vi "Get Fault States.vi"(8 "error in (no error)":errorcluster, 11 "FIU Board Ref in":T1 format="%.0x") -> (0 "error out":errorcluster, 1 "Ordered Fault Channels":T1[](array[typedef]) format="%.0x", 2 "Fault States":T2[](array[typedef]), 3 "FIU Board Ref out":T1 format="%.0x")   [LabVIEW 2014, in "SLSC configuration System Explorer.lvlib"]
doc: "Orders the fault channels and gets the current fault states of a single FIU board."
uses:
  SLSC configuration System Explorer.lvlib
  <vilib>/NI Veristand/Custom Device API/Custom Device Item Ref.ctl
  Example/FIU Board/Fault State.ctl
  Shared/Constants.vi
  <vilib>/NI Veristand/Custom Device API/Get Item Property (U16).vi
  <vilib>/NI Veristand/Custom Device API/Custom Device API.lvlib
  Shared/SLSC configuration Shared.lvlib
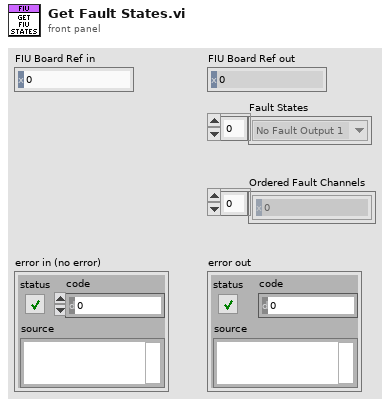
[diagram p1: front panel]
types:
  T1 = typedef "Custom Device API.lvlib/Custom Device Item Ref.ctl" = u64
  T2 = typedef "SLSC configuration Shared.lvlib/Fault State.ctl" = enum8{"No Fault Output 1", "Open Circuit 100 Hz", "Ground 100 Hz", "Open Circuit", "Ground", "Fail Rail 1", "Fail Rail 2", "No Fault Output 2"}
  T3 = typedef "Custom Device API.lvlib/Custom Device Channel.ctl" = cluster{"Type":T4, "Units":string, "Default Value":dbl, "Faultable":bool, "Scalable":bool}
  T4 = typedef "Custom Device API.lvlib/Custom Device Channel Type.ctl" = enum16{"Input", "Output"}
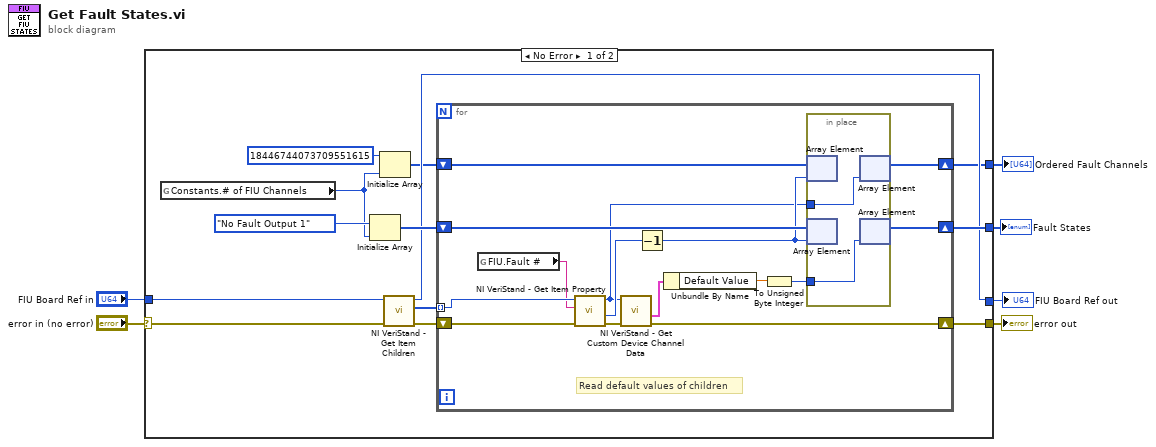
[diagram p0: block diagram]
diagram:
  n1 = case shown="No Error" "error in (no error)" {
    selector: "error in (no error)" -> [w12 w37]
    tunnel: "FIU Board Ref in" -> [w17 w38]
    tunnel: [w16 w37] -> w5
    tunnel: [w13 _] -> w4
    tunnel: [w11 w38] -> w2
    tunnel: [w7 _] -> w1
    frame No Error {
      n2 = global read "Constants.vi" "Constants.# of FIU Channels"() -> (w9:u8)
      n3 = Initialize Array(Fault_State."No Fault Output 1" ("dimension size"), w9) -> (w19:T2[])
      n4 = Initialize Array(T1 18446744073709551615 ("Item Ref out"), w9) -> (w8:T1[])
      n5 = call <vilib>:"NI VeriStand - Get Item Children.vi"("error in (no error)"=w12, "Item Ref in"=w17) -> ("error out"=w15:errorcluster, "Child Refs"=w14:T1[], "Item Ref out"=w11:T1)  [unwired: 6 in, 1 out]
      n6 = for {
        tunnel: w14 -> [w34] mode=indexing
        shift-right: [w26] -> w16
        shift-left: w15 -> [w32]
        shift-right: [w24] -> w13
        shift-left: w19 -> [w27]
        shift-right: [w20] -> w7
        shift-left: w8 -> [w23]
        # "Read default values of children"
        n7 = global read "Constants.vi" "FIU.Fault #"() -> (w33:string)
        n8 = call-poly <vilib>:"NI VeriStand - Get Item Property.vi"("error in (no error)"=w32, "Property Name"=w33, "Item Ref in"=w34) -> ("error out"=w30:errorcluster, "Value"=w31:u16, "Item Ref out"=w21:T1)  [unwired: 5 in, 1 out]
        n9 = call <vilib>:"NI VeriStand - Get Custom Device Channel Data.vi"("error in (no error)"=w30, "Channel Ref in"=w21) -> ("error out"=w26:errorcluster, "Channel"=w29:T3)  [unwired: 4 in, 4 out]
        n10 = Decrement(x=w31) -> (x-1=w22:u16)
        n11 = Unbundle By Name(w29) -> ("Default Value"=w28:dbl)
        n12 = To Unsigned Byte Integer(number=w28) -> (unsigned 8bit integer=w25:u8)
        n13 = in-place {
          in-place-border: w25 -> [w36]
          in-place-border: w21 -> [w35]
          n14 = in-place-array #1(w23, w22) -> ()  [unwired: 1 out]
          n15 = in-place-array #2(w27, w22) -> ()  [unwired: 1 out]
          n16 = in-place-array #1(w35) -> (w20:T1[])  [unwired: 1 out]
          n17 = in-place-array #2(w36) -> (w24:T2[])  [unwired: 1 out]
        }
      }
    }
    frame Error {
    }
  }
  "error out" <- w5
  "Fault States" <- w4
  "FIU Board Ref out" <- w2
  "Ordered Fault Channels" <- w1
